vi "Convert FPS to RPM.vi"(5 "RevMotor/RevWheel":dbl=6.67 format="%#_13g", 7 "Wheel Diameter (in)":dbl=4.0 format="%#_13g", 11 "Translation Speed (ft/s)":dbl) -> (3 "Motor Speed (RPM) Out":dbl)   [LabVIEW 2020, in "SwerveDrive_ACT_ts.lvlib"]
uses:
  SwerveDrive_ACT_ts.lvlib
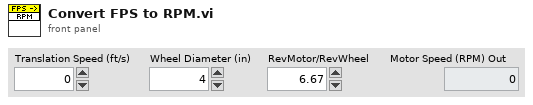
[diagram p1: front panel]
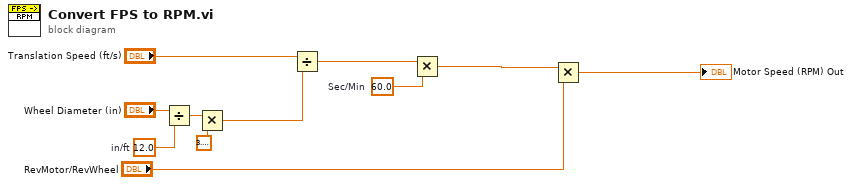
[diagram p0: block diagram]
diagram:
  w3 = 60.0  # Sec/Min
  w10 = 12.0  # in/ft
  n1 = Divide(x="Wheel Diameter (in)", y=w10) -> (x/y=w8:dbl)
  n2 = Multiply(x=w8, y=3.141592653589793) -> (x*y=w7:dbl)
  n3 = Divide(x="Translation Speed (ft/s)", y=w7) -> (x/y=w5:dbl)
  n4 = Multiply(x=w5, y=w3) -> (x*y=w4:dbl)
  n5 = Multiply(x=w4, y="RevMotor/RevWheel") -> (x*y=→"Motor Speed (RPM) Out":dbl)
